vi "demo.vi"() -> ()   [LabVIEW 2020]
panel:
  out "DEMO1 > DEMO2?":bool
  in  "y_2":dbl
  in  "Slide":dbl(slide) scale=20.0..50.0
  out "C = sqrt(A^2 + B^2)":dbl
  in  "B":dbl
  in  "A":dbl
  in  "y":dbl
  in  "Knob":dbl(knob) scale=20.0..50.0
  # "DEMO1"
  # "Right triangle Hypotenuse"
  # "DEMO2"
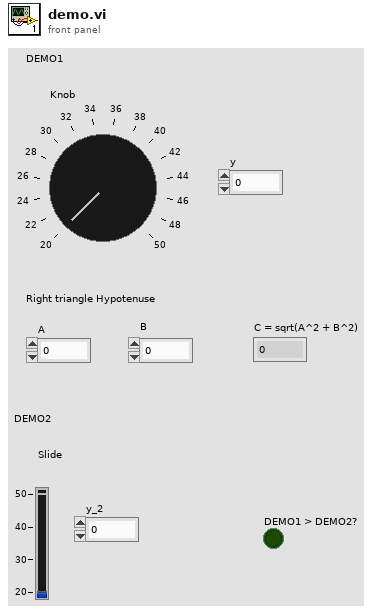
[diagram p1: front panel]
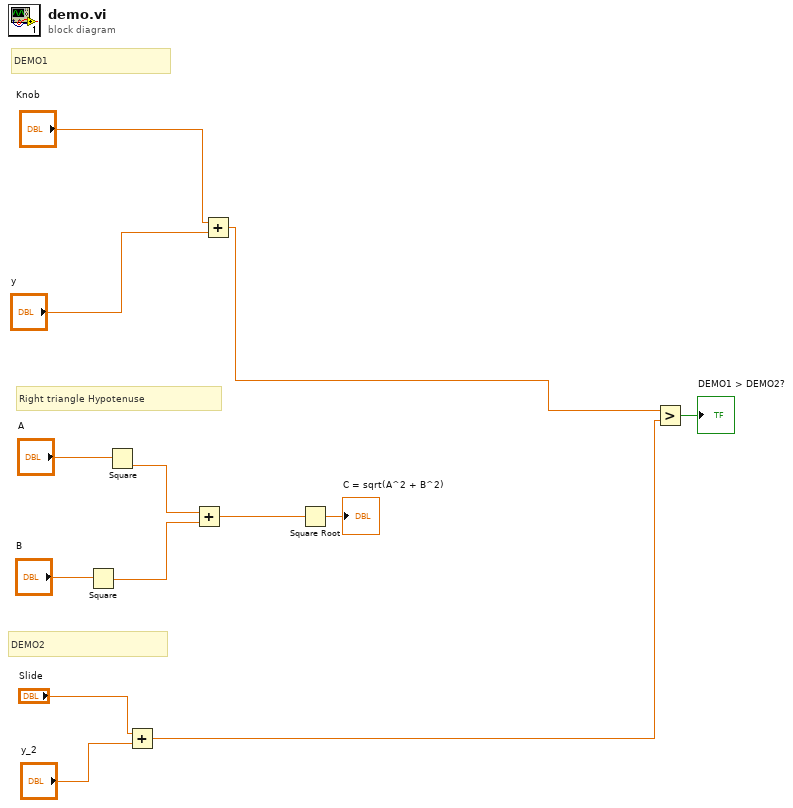
[diagram p0: block diagram]
diagram:
  # "DEMO2"
  # "Right triangle Hypotenuse"
  # "DEMO1"
  n1 = Square(x="B") -> (x^2=w8:dbl)
  n2 = Square(x="A") -> (x^2=w9:dbl)
  n3 = Add(x="Slide", y="y_2") -> (x+y=w2:dbl)
  n4 = Add(x=w9, y=w8) -> (x+y=w7:dbl)
  n5 = Add(x="Knob", y="y") -> (x+y=w3:dbl)
  n6 = Square Root(x=w7) -> (sqrt(x)=→"C = sqrt(A^2 + B^2)":dbl)
  n7 = Greater?(x=w3, y=w2) -> (0:→"DEMO1 > DEMO2?":bool)
